vi "Measure.vi"(8 "error in":errorcluster, 11 "AnalogInput in":refnum<class "AnalogInput.lvclass">) -> (0 "error out":errorcluster, 3 "AnalogInput out":refnum<class "AnalogInput.lvclass">)   [LabVIEW 2019, in "AnalogInput.lvlib" / "AnalogInput.lvclass"]
uses:
  Library/AnalogInput.lvclass
  builds/Instruments/Instruments.lvlibp/Library/Instruments.lvclass
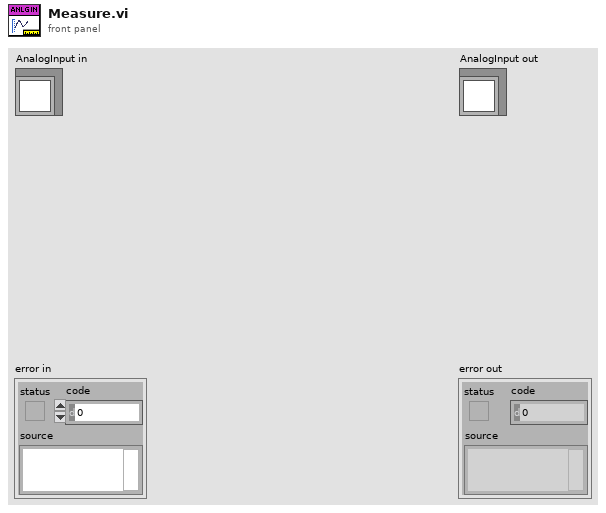
[diagram p1: front panel]
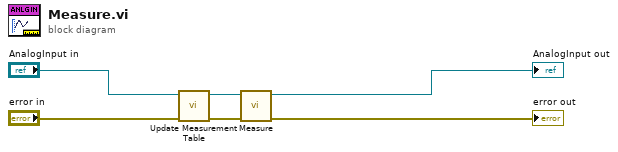
[diagram p0: block diagram]
diagram:
  n1 = call "Update Measurement Table.vi"("error in (no error)"="error in", "AnalogInput in"="AnalogInput in") -> ("error out"=w2:errorcluster, "AnalogInput out"=w1:refnum<class "AnalogInput.lvclass">)  [unwired: 8 in]
  n2 = call-parent "Measure.vi"("error in"=w2, "Instruments in"=w1) -> ("error out"=→"error out":errorcluster, "Instruments out"=→"AnalogInput out":refnum<class "AnalogInput.lvclass">)  [unwired: 8 in]
